vi "Start into stacking.vi"(1 "ふ计":i32, 5 "KNR in":T2, 9 "Circles (Shape Detection 1) 2":T1(array[cluster]) {"Position"."Y" format="%.2f"; "Position"."X" format="%.2f"}, 11 "Error":errorcluster) -> (2 "Y軸補正":i32, 3 "X":i32, 4 "最終堆疊版":bool[][](array[boolean]), 6 "KNR out":T2, 8 "底盤T數":i32, 10 "旋轉數":i32, 12 "配對數":i32, 13 "層數":i32, 14 "Y":i32, 15 "error out":errorcluster)   [LabVIEW 2013]
uses:
  <userlib>/_FPGA Interface Advanced Tools/FPGA Interface Base/FPGA Interface Base.lvclass
  <userlib>/KNR OS 3.0 LabVIEW Toolkit/Type Definition/Resource.ctl
  <userlib>/KNR OS 3.0 LabVIEW Toolkit/Type Definition/KNR3 Reference.ctl
panel:
  out "配對積木":bool[][](array[boolean])
  out "最終排數":i32
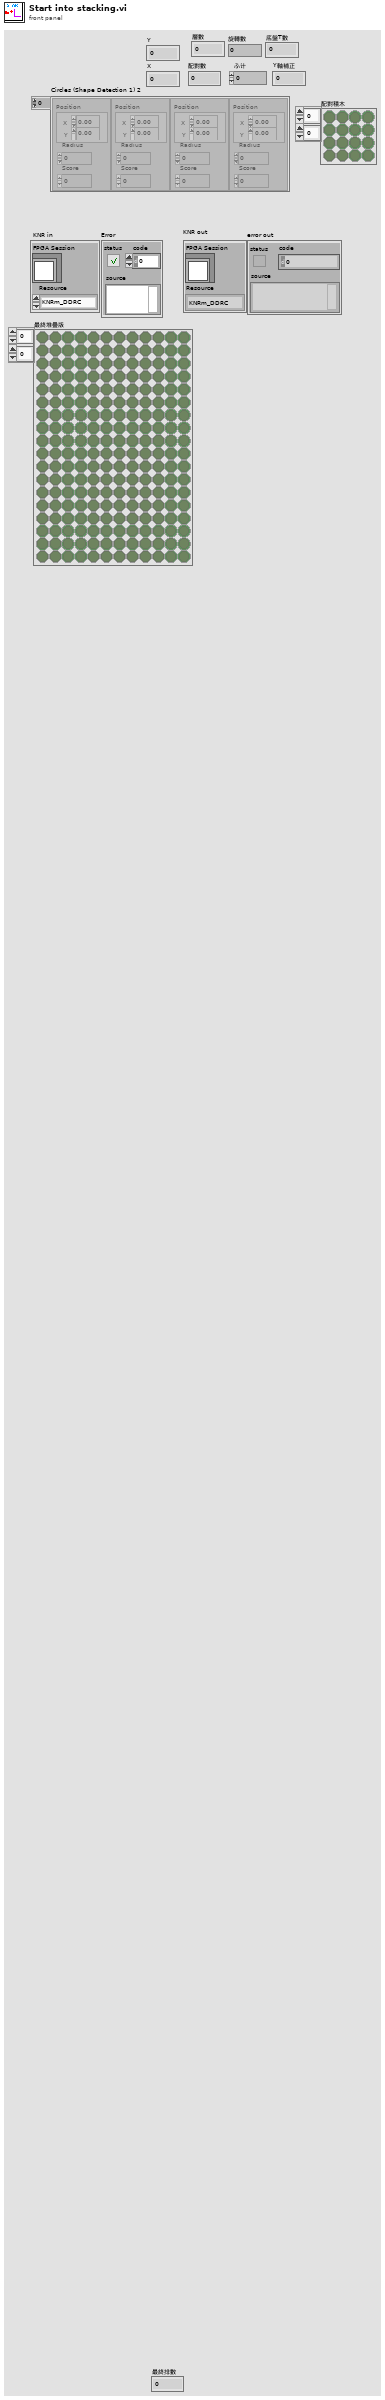
[diagram p1: front panel]
types:
  T1 = cluster{"Position":cluster{"X":sgl, "Y":sgl}, "Radius":dbl, "Score":dbl}[]
  T2 = typedef "KNR3 Reference.ctl" = cluster{"FPGA Session":refnum<class "FPGA Interface Base.lvclass">, "Resource":T3}
  T3 = typedef "Resource.ctl" = enum16{"KNRm_DDRC", "KNRm_DDDD", "KNRm_DDDR", "KNRm_DDDC", "KNR"}
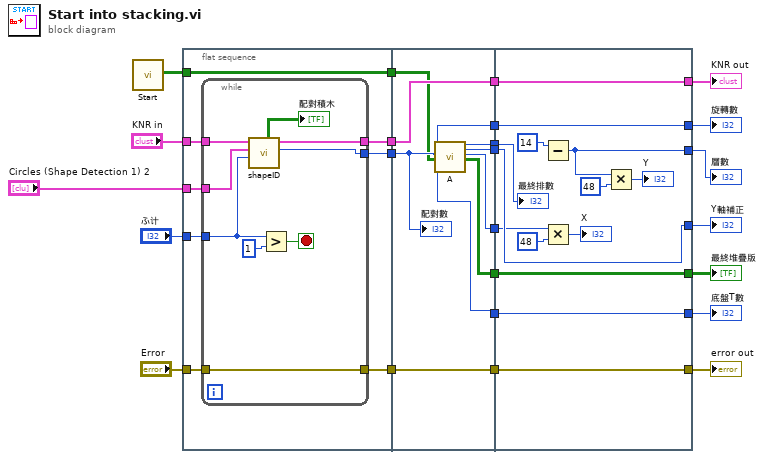
[diagram p0: block diagram]
diagram:
  n1 = call "Start.vi"() -> ("初始堆疊版"=w11:bool[][])  [unwired: 11 in]
  n2 = flat-sequence {
    tunnel: [w32] -> w24
    tunnel: w11 -> [w31]
    tunnel: [w31] -> w23
    tunnel: "KNR in" -> [w30]
    tunnel: "Error" -> [w29]
    tunnel: [w28] -> w20
    tunnel: [w27] -> w15
    tunnel: "Circles (Shape Detection 1) 2" -> [w26]
    tunnel: "ふ计" -> [w25]
    tunnel: w24 -> [w44]
    tunnel: w23 -> [w42]
    tunnel: w20 -> [w51]
    tunnel: [w51] -> w17
    tunnel: [w50] -> w16
    tunnel: w15 -> [w50]
    tunnel: [w49] -> w10
    tunnel: [w48] -> w9
    tunnel: [w47] -> w7
    tunnel: [w46] -> w6
    tunnel: [w45] -> w4
    tunnel: [w43] -> w2
    tunnel: [w60] -> w18
    tunnel: [w65] -> w19
    tunnel: w17 -> [w65]
    tunnel: w16 -> [w60]
    tunnel: [w58] -> w12
    tunnel: w10 -> [w57]
    tunnel: w9 -> [w56]
    tunnel: [w56] -> w8
    tunnel: w7 -> [w55]
    tunnel: w6 -> [w54]
    tunnel: [w54] -> w5
    tunnel: w4 -> [w53]
    tunnel: [w53] -> w3
    tunnel: w2 -> [w52]
    tunnel: [w52] -> w1
    frame #0 {
      n3 = while {
        tunnel: [w39] -> w32
        tunnel: w30 -> [w37]
        tunnel: w29 -> [w36]
        tunnel: [w38] -> w28
        tunnel: [w36] -> w27
        tunnel: w26 -> [w35]
        tunnel: w25 -> [w34]
        stop <- w40 stop-if-true
        n4 = call "shapeID.vi"("Nb Circles (Circle Detection 1)"=w34, "Circles (Shape Detection 1)"=w35, "KNR in"=w37) -> ("配對數"=w39:i32, "KNR out"=w38:T2, "配對積木"=→"配對積木":bool[][])  [unwired: 5 in, 1 out]
        n5 = Greater?(x=w34, y=1) -> (0:w40:bool)
      }
    }
    frame #1 {
      n6 = call "A.vi"("積木種類"=w44, "初始進入"=w42) -> ("旋轉數"=w43:i32, "底盤T數"=w45:i32, "end"=w49:i32, "Y軸補正"=w48:i32, "移動位置"=w47:i32, "最終堆疊版"=w46:bool[][])  [unwired: 9 in, 3 out]
      "配對數" <- w44
    }
    frame #2 {
      n7 = Subtract(x=14) -> (x-y=w58:i32)  [unwired: 1 in]
      n8 = Multiply(x=w55, y=48) -> (x*y=→"X":i32)
      n9 = Multiply(x=w58, y=48) -> (x*y=→"Y":i32)
      "最終排數" <- w57
    }
  }
  "最終堆疊版" <- w5
  "KNR out" <- w19
  "error out" <- w18
  "旋轉數" <- w1
  "層數" <- w12
  "底盤T數" <- w3
  "Y軸補正" <- w8
